vi "Xeryon Read COM port number.vi"() -> (1 "COM-port":string)   [LabVIEW 2019]
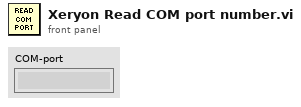
[diagram p1: front panel]
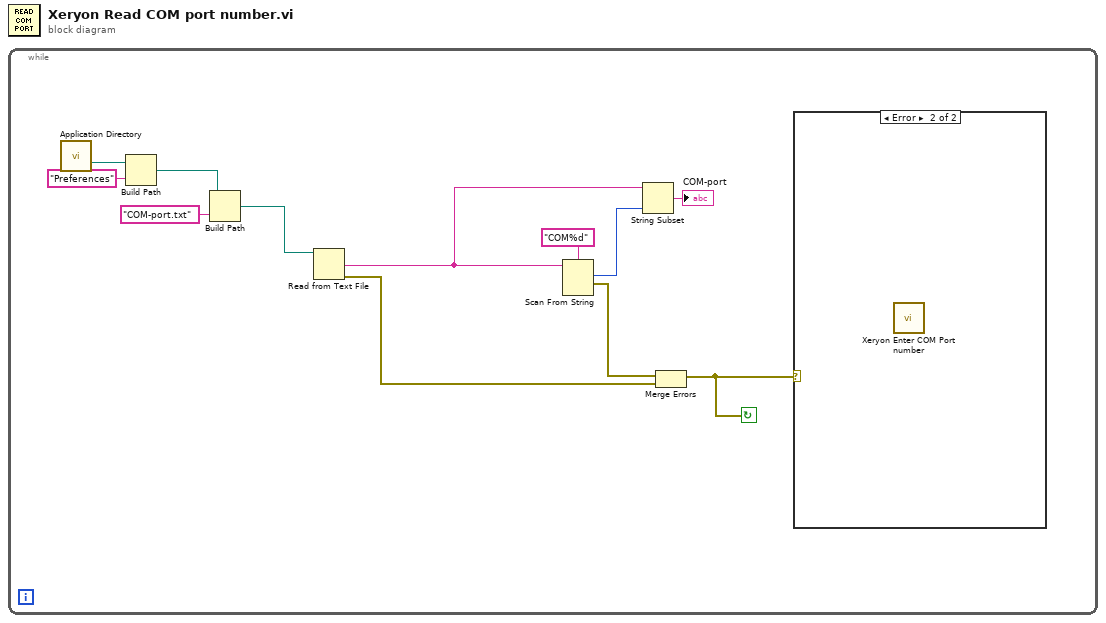
[diagram p0: block diagram]
diagram:
  n1 = while {
    stop <- w1 continue-if-true
    n2 = call <vilib>:"Application Directory.vi"() -> ("Application Directory"=w5:path)
    n3 = Build Path(base path=w5, name or relative path="Preferences") -> (appended path=w7:path)
    n4 = Build Path(base path=w7, name or relative path="COM-port.txt") -> (appended path=w4:path)
    n5 = Read from Text File(file (use dialog)=w4) -> (text=w11:string, error out=w2:errorcluster)  [unwired: 3 in, 2 out]
    n6 = Scan From String(format string="COM%d", input string=w11) -> (offset past scan=w10:u32, error out=w3:errorcluster)  [unwired: 4 in, 1 out]
    n7 = String Subset(string=w11, length (rest)=w10) -> (substring=→"COM-port":string)  [unwired: 1 in]
    n8 = Merge Errors(w3, w2) -> (w1:errorcluster)
    n9 = case shown="Error" w1 {
      frame No Error {
      }
      frame Error {
        n10 = call "Xeryon Enter COM Port number.vi"() -> ()  [unwired: 6 in]
      }
    }
  }
